vi "Read Cipher.vi"(11 "Message Stream in":refnum<class "Message Stream.lvclass">) -> (2 "Cipher.lvclass":refnum<class "Cipher.lvclass">)   [LabVIEW 2020, in "Message Stream.lvclass"]
doc: "Use this accessor to obtain the cipher currently being used by this stream."
uses:
  Message Stream.lvclass
  Cipher/Cipher.lvclass
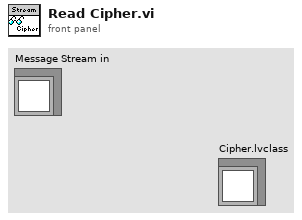
[diagram p1: front panel]
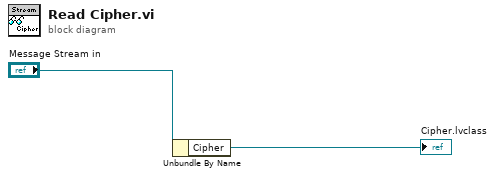
[diagram p0: block diagram]
diagram:
  n1 = Unbundle By Name("Message Stream in") -> ("Cipher"=→"Cipher.lvclass":refnum<class "Cipher.lvclass">)
